vi "scan position (SubVI).vi"(6 "字符串":string, 10 "config":T1={"initialize"="", "6221"={"6221 Resource"="GPIB0::24::INSTR", "Delta status"=FALSE}, "7001"={"Ch"=FALSE}, "SR830+6221"={"source"=0, "阻抗"=0.0, "量程入 4"=0, "量程入 3"=0, "量程入 2"=0, "量程入 1"=0, "电流"=0.0, "SR830 2"=FALSE, "SR830 3"=FALSE, "SR830 4"=FALSE, "SR830 1"=FALSE, "VISA 1"="", "VISA 2"="", "VISA 3"="", "VISA 4"="", "量程"=enum."量程每次测量会判定"}, "2400"={"2400"=FALSE, "VISA"=""}, "ch"={"ch str"="", "ch1"=FALSE, "ch2"=FALSE, "布尔"=FALSE}, "数据文件路径"=path "", "log"={"log路径"=path "", "log interval"=0.0}, "Instrument"={"335 Resource"="GPIB0::24::INSTR", "Input (0:A)"=0, "Instrument Type"=3, "quantum design"=refnum, "Heater Output (1:1)"=1, "semaphore"=refnum, "TCP master instance"=refnum, "335 Status"=refnum, "M24C Resource"="GPIB0::24::INSTR", "4G supply"="GPIB0::24::INSTR", "Temp Status 24C"=refnum, "4g supply status"=refnum}, "Aborting"=refnum} {"Instrument"."Input (0:A)" items=["A", "B"]; "Instrument"."Instrument Type" items=["PPMS", "VersaLab", "DynaCool", "SVSM", "Lakeshore335", "PPMS-Rotate"]; "Instrument"."Heater Output (1:1)" items=["1"=1, "2"=2]; "SR830+6221"."source" items=["SR830 1", "SR830 2", "SR830 3", "SR830 4"]}, 11 "队列输入":refnum<queue>) -> (0 "错误输出":errorcluster, 3 "输出簇":T1={"initialize"="", "6221"={"6221 Resource"="GPIB0::24::INSTR", "Delta status"=FALSE}, "7001"={"Ch"=FALSE}, "SR830+6221"={"source"=0, "阻抗"=0.0, "量程入 4"=0, "量程入 3"=0, "量程入 2"=0, "量程入 1"=0, "电流"=0.0, "SR830 2"=FALSE, "SR830 3"=FALSE, "SR830 4"=FALSE, "SR830 1"=FALSE, "VISA 1"="", "VISA 2"="", "VISA 3"="", "VISA 4"="", "量程"=enum."量程每次测量会判定"}, "2400"={"2400"=FALSE, "VISA"=""}, "ch"={"ch str"="", "ch1"=FALSE, "ch2"=FALSE, "布尔"=FALSE}, "数据文件路径"=path "", "log"={"log路径"=path "", "log interval"=0.0}, "Instrument"={"335 Resource"="GPIB0::24::INSTR", "Input (0:A)"=0, "Instrument Type"=3, "quantum design"=refnum, "Heater Output (1:1)"=1, "semaphore"=refnum, "TCP master instance"=refnum, "335 Status"=refnum, "M24C Resource"="GPIB0::24::INSTR", "4G supply"="GPIB0::24::INSTR", "Temp Status 24C"=refnum, "4g supply status"=refnum}, "Aborting"=refnum} {"Instrument"."Input (0:A)" items=["A", "B"]; "Instrument"."Instrument Type" items=["PPMS", "VersaLab", "DynaCool", "SVSM", "Lakeshore335", "PPMS-Rotate"]; "Instrument"."Heater Output (1:1)" items=["1"=1, "2"=2]; "SR830+6221"."source" items=["SR830 1", "SR830 2", "SR830 3", "SR830 4"]})   [LabVIEW 2019, in "SubVI.lvlib"]
uses:
  SubVI.lvlib
  config.ctl
  <vilib>/NI/Modbus Library/API/Master/Modbus Master.lvclass
  Instrument.ctl
  lib/QDInstrument.dll
  335 state.ctl
panel:
  # "(真是通道1，假是通道2)"
  # "(真是通道1，假是通道2)"
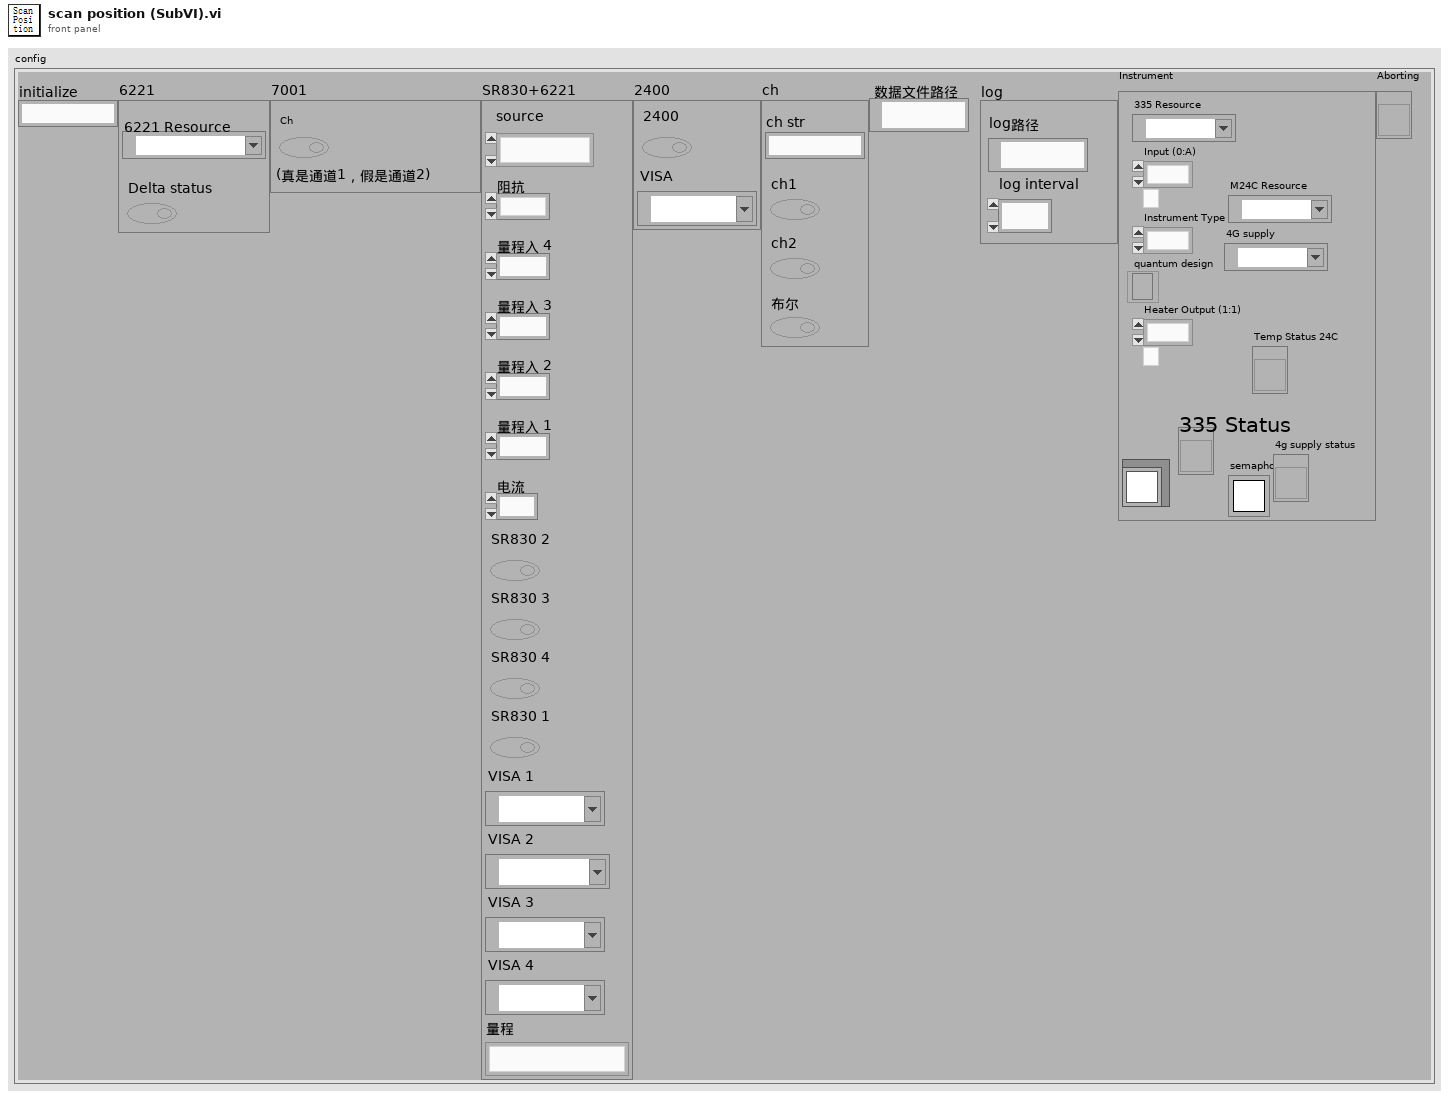
[diagram p1: front panel]
types:
  T1 = typedef "config.ctl" = cluster{"initialize":string, "6221":cluster{"6221 Resource":refnum<visa-resource-name>, "Delta status":bool}, "7001":cluster{"Ch":bool}, "SR830+6221":cluster{"source":u16, "阻抗":dbl, "量程入 4":i32, "量程入 3":i32, "量程入 2":i32, "量程入 1":i32, "电流":dbl, "SR830 2":bool, "SR830 3":bool, "SR830 4":bool, "SR830 1":bool, "VISA 1":refnum<visa-resource-name>, "VISA 2":refnum<visa-resource-name>, "VISA 3":refnum<visa-resource-name>, "VISA 4":refnum<visa-resource-name>, "量程":enum16{"量程每次测量会判定", "量程不变为设定值"}}, "2400":cluster{"2400":bool, "VISA":refnum<visa-resource-name>}, "ch":cluster{"ch str":string, "ch1":bool, "ch2":bool, "布尔":bool}, "数据文件路径":path, "log":cluster{"log路径":path, "log interval":dbl}, "Instrument":T2, "Aborting":refnum<vi>}
  T2 = typedef "Instrument.ctl" = cluster{"335 Resource":refnum<visa-resource-name>, "Input (0:A)":u16, "Instrument Type":i32, "quantum design":refnum<k24>, "Heater Output (1:1)":u16, "semaphore":T3, "TCP master instance":refnum<class "Modbus Master.lvclass">, "335 Status":refnum<vi>, "M24C Resource":refnum<visa-resource-name>, "4G supply":refnum<visa-resource-name>, "Temp Status 24C":refnum<vi>, "4g supply status":refnum<vi>}
  T3 = typedef "Semaphore RefNum" = refnum<k1>
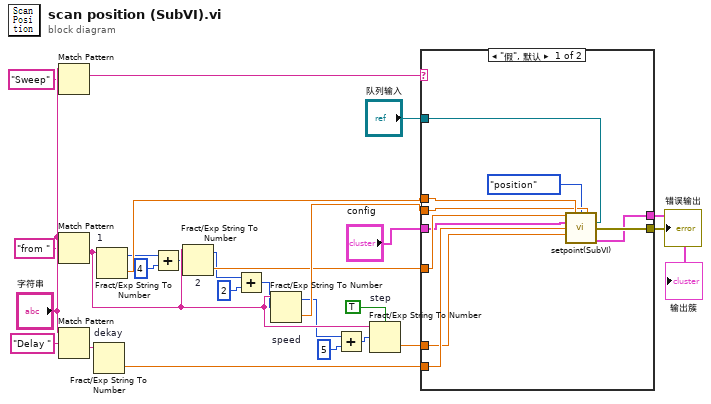
[diagram p0: block diagram]
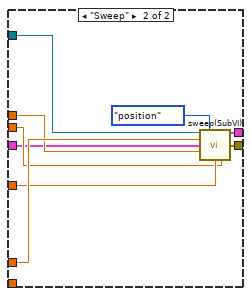
[diagram p2: hidden frame]
diagram:
  n1 = Match Pattern(string="字符串", regular expression="Sweep" ("正则表达式")) -> (match substring=w15:string)  [unwired: 1 in, 3 out]
  n2 = Match Pattern(string="字符串", regular expression="from " ("正则表达式")) -> (after substring=w19:string)  [unwired: 1 in, 3 out]
  n3 = Match Pattern(string="字符串", regular expression="Delay " ("正则表达式")) -> (after substring=w18:string)  [unwired: 1 in, 3 out]
  n4 = Fract/Exp String To Number "dekay"(string=w18) -> (number=w21:dbl)  [unwired: 3 in, 1 out]
  n5 = Fract/Exp String To Number "1"(string=w19) -> (offset past number=w4:i32, number=w25:dbl)  [unwired: 3 in]
  n6 = Add(x=w4, y=4) -> (x+y=w6:i32)
  n7 = Fract/Exp String To Number "2"(string=w19, offset=w6) -> (offset past number=w7:i32, number=w20:dbl)  [unwired: 2 in]
  n8 = Add(x=w7, y=2) -> (x+y=w9:i32)
  n9 = Fract/Exp String To Number "speed"(string=w19, offset=w9) -> (offset past number=w10:i32, number=w23:dbl)  [unwired: 2 in]
  n10 = Add(x=w10, y=5) -> (x+y=w12:i32)
  n11 = Fract/Exp String To Number "step"(use system decimal point (T)=TRUE ("使用系统小数点(T)"), string=w19, offset=w12) -> (number=w22:dbl)  [unwired: 1 in, 1 out]
  n12 = case shown="\"假\", 默认" w15 {
    tunnel: w20 -> [w36 w41]
    tunnel: w21 -> [w33 _]
    tunnel: w22 -> [w32 w43]
    tunnel: w23 -> [w31 w40]
    tunnel: "队列输入" -> [w34 w45]
    tunnel: w25 -> [w35 w42]
    tunnel: [w29 w39] -> w26
    tunnel: "config" -> [w28 w38]
    tunnel: [w27 w37] -> w1
    frame "假", Default {
      n13 = call "setpoint(SubVI).vi"("Filed 2"=w36, "Field"=w35, "类型"=enum16{"temp", "field", "position"}."position", "Rate/speed"=w31, "输出簇 2"=w28, "data"=w34, "Delay"=w33, "steps number"=w32) -> ("错误输出"=w29:errorcluster, "输出簇"=w27:T1)  [unwired: 6 in]
    }
    frame "Sweep" {
      n14 = call "sweep(SubVI).vi"("data"=w45, "类型"=enum16{"temp", "field", "position"}."position", "steps number"=w43, "簇"=w38, "Field"=w42, "Field 2"=w41, "Rate、speed"=w40) -> ("输出簇"=w37:T1, "错误输出"=w39:errorcluster)  [unwired: 7 in]
    }
  }
  "错误输出" <- w26
  "输出簇" <- w1
